vi "Inverse.vi"() -> ()   [LabVIEW 2018]
doc: "Use this template to build a VI to use as a subVI."
uses:
  <vilib>/vision/NI_Vision_Development_Module.lvlib
panel:
  out "Src":T1(plugin-control)
  out "Dst":T1(plugin-control)
  # ":: MVi Framework V1.0 ::\nAuthor:Gaoke Yang\nEmail: gaoke.yang@yahoo.com\nWeb: www.mvicontrol.com\nCopyright (C) 2015, MVI Technologies All Rights Reserved"
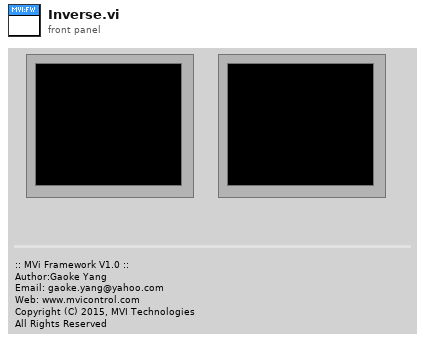
[diagram p1: front panel]
types:
  T1 = typedef "IMAQ Image.ctl" = refnum<image>
  T2 = typedef "Image Type" = u32
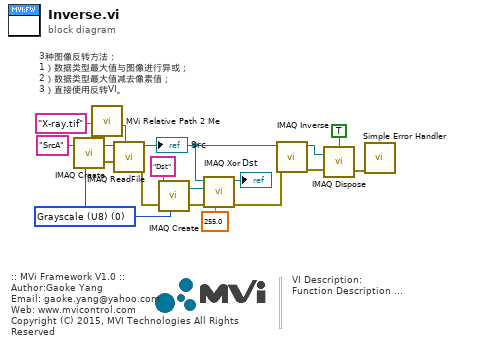
[diagram p0: block diagram]
diagram:
  w1 = T2 0 items=["Grayscale (U8)", "Grayscale (I16)", "Grayscale (SGL)", "Complex (CSG)", "RGB (U32)", "HSL (U32)", "RGB (U64)", "Grayscale (U16)"] ("Image Type")
  # "3种图像反转方法：\n1）数据类型最大值与图像进行异或；\n2）数据类型最大值减去像素值；\n3）直接使用反转VI。"
  # "VI Description:\nFunction Description ..."
  # ":: MVi Framework V1.0 ::\nAuthor:Gaoke Yang\nEmail: gaoke.yang@yahoo.com\nWeb: www.mvicontrol.com\nCopyright (C) 2015, MVI Technologies All Rights Reserved"
  n1 = call "IMAQ Create"("Image Name"="SrcA" ("name or relative path"), "Image Type"=w1) -> ("New Image"=w12:T1, "error out"=w11:errorcluster)  [unwired: 2 in, 1 out]
  n2 = call "MVi Relative Path 2 Me.vi"("Relative Path"="X-ray.tif" ("name or relative path")) -> ("Appended Dir"=w14:path)  [unwired: 5 in, 1 out]
  n3 = call "IMAQ ReadFile"("File Path"=w14, "error in (no error)"=w11, "Image"=w12) -> ("error out"=w10:errorcluster, "Image Out"=w6:T1)  [unwired: 4 in, 3 out]
  "Src" <- w6
  n4 = call "IMAQ Create"("Image Name"="Dst" ("name or relative path"), "Image Type"=w1, "error in (no error)"=w10) -> ("New Image"=w5:T1, "error out"=w4:errorcluster)  [unwired: 1 in, 1 out]
  n5 = call "IMAQ Xor"("Constant"=255.0, "error in (no error)"=w4, "Image Dst"=w5, "Image Src A"=w6) -> ("error out"=w8:errorcluster, "Image Dst Out"=→"Dst":T1)  [unwired: 6 in]
  n6 = call "IMAQ Inverse"("error in (no error)"=w8, "Image Src"=w6) -> ("error out"=w7:errorcluster, "Image Dst Out"=w3:T1)  [unwired: 8 in]
  n7 = call "IMAQ Dispose"("All Images? (No)"=TRUE, "Image"=w3, "error in (no error)"=w7) -> ("error out"=w15:errorcluster)  [unwired: 3 out]
  n8 = call <vilib>:"Simple Error Handler.vi"("error in (no error)"=w15) -> ()  [unwired: 1 in, 8 out]
